vi "Format and Log Text.vi"(7 "Debug Level":T1=enum."INFO", 8 "error in (no error)":errorcluster, 10 "Log Text":string, 11 "Logger in":refnum<class "Logger.lvclass">) -> (0 "error out":errorcluster, 2 "Log Output":string, 3 "Logger out":refnum<class "Logger.lvclass">)   [LabVIEW 2020, in "LV Logging.lvlib" / "Logger.lvclass"]
uses:
  Logger.lvclass
  Logger.lvclass/Logger.ctl
  LV Logging.lvlib
  Type Defs/Debug Level.ctl
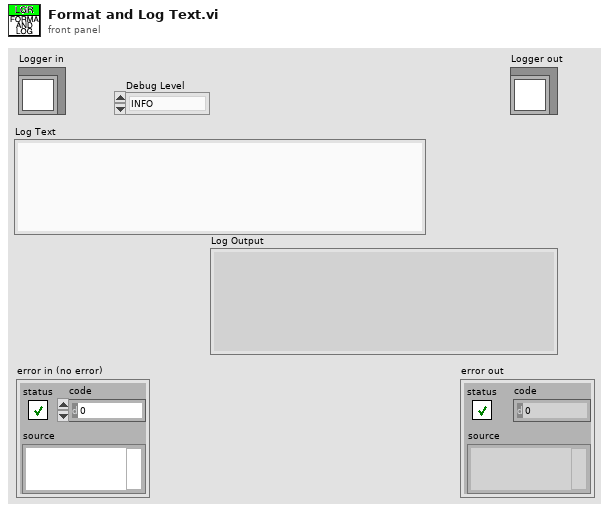
[diagram p1: front panel]
types:
  T1 = typedef "LV Logging.lvlib/Debug Level.ctl" = enum16{"DEBUG", "INFO", "WARN", "ERROR", "FATAL"}
  T2 = enum16{"Init", "Get Logger", "Register Sink", "Set Global Debug Level", "Get Sinks", "Get Global Debug Level"}
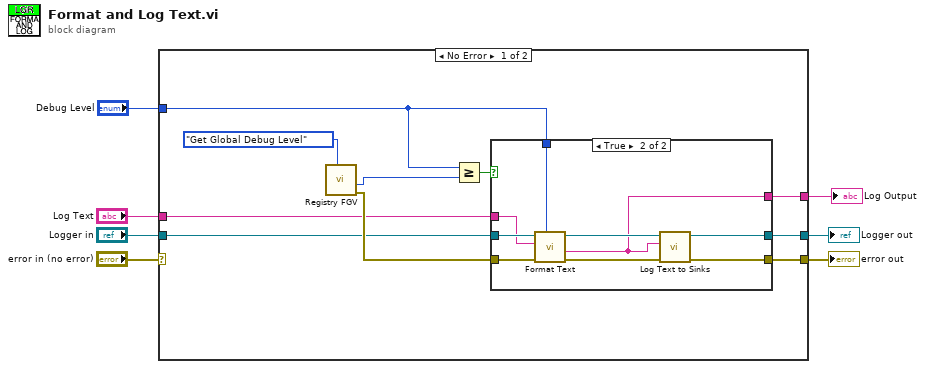
[diagram p0: block diagram]
diagram:
  n1 = case shown="No Error" "error in (no error)" {
    selector: "error in (no error)" -> [_ w30]
    tunnel: [w12 w30] -> w6
    tunnel: [w13 w29] -> w4
    tunnel: "Logger in" -> [w14 w29]
    tunnel: [w11 _] -> w3
    tunnel: "Log Text" -> [w10 _]
    tunnel: "Debug Level" -> [w8 _]
    frame No Error {
      n2 = call "Registry FGV.vi"("State (Get Logger)"=T2."Get Global Debug Level") -> ("error out"=w17:errorcluster, "Debug Level out"=w9:T1)  [unwired: 7 in, 2 out]
      n3 = Greater Or Equal?(x=w8, y=w9) -> (x >= y?=w15:bool)
      n4 = case shown="True" w15 {
        tunnel: [w18 w26] -> w13
        tunnel: [w19 w25] -> w12
        tunnel: [_ w24] -> w11
        tunnel: w17 -> [w19 w23]
        tunnel: w14 -> [w18 w22]
        tunnel: w10 -> [_ w21]
        tunnel: w8 -> [_ w20]
        frame False {
        }
        frame True {
          n5 = call "Format Text.vi"("Debug Level"=w20, "error in (no error)"=w23, "Log Text"=w21, "Logger in"=w22) -> ("error out"=w28:errorcluster, "Log Output"=w24:string, "Logger out"=w27:refnum<class "Logger.lvclass">)  [unwired: 5 in]
          n6 = call "Log Text to Sinks.vi"("error in (no error)"=w28, "Log Text"=w24, "Logger in"=w27) -> ("error out"=w25:errorcluster, "Logger out"=w26:refnum<class "Logger.lvclass">)  [unwired: 7 in]
        }
      }
    }
    frame Error {
    }
  }
  "error out" <- w6
  "Logger out" <- w4
  "Log Output" <- w3
